vi "Optitrack Global.vi"() -> ()   [LabVIEW 2021]
panel:
  in  "Position Offset":dbl[](array[numeric]) format="%.2f"
  in  "Position XYZ":dbl[](array[numeric]) format="%.2f"
  in  "Position Array":dbl[][](array[numeric])
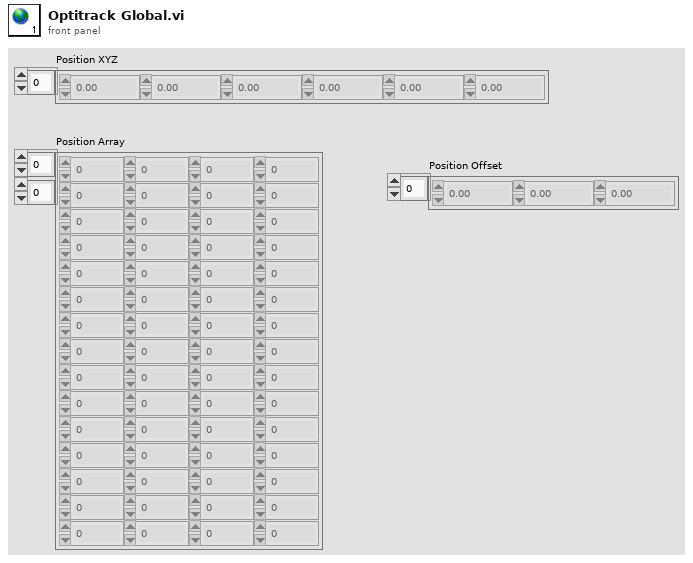
[diagram p1: front panel]
diagram:
